vi "Configure voltage read.vi"(6 "error in":errorcluster, 8 "Range":string, 9 "VISA resource name":refnum<visa-resource-name>) -> (0 "error out":errorcluster, 3 "VISA resource name out":refnum<visa-resource-name>)   [LabVIEW 2023, in "Aim TTi 1908P DMM.lvlib"]
uses:
  Aim TTi 1908P DMM.lvlib
  34c442d0-076a-446d-8d09-49ed1551a703.vi
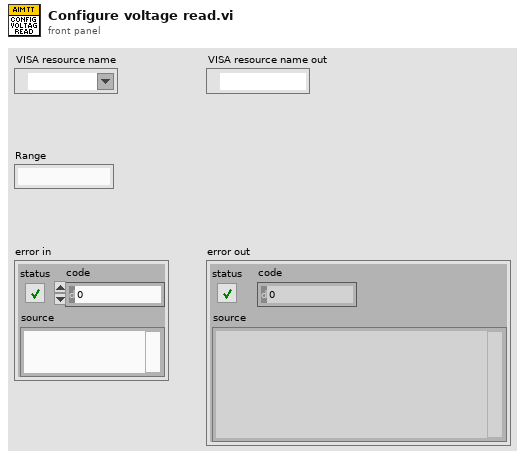
[diagram p1: front panel]
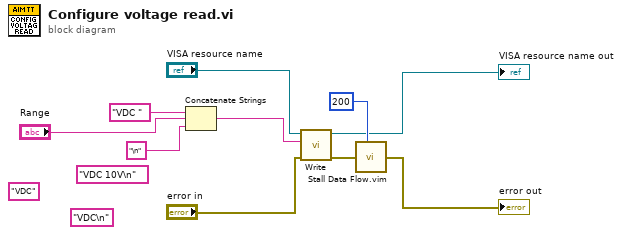
[diagram p0: block diagram]
diagram:
  (unwired) "VDC\n" ("Data to write")
  (unwired) "VDC 10V\n" ("Data to write")
  (unwired) "VDC" ("Data to write")
  n1 = Concatenate Strings("VDC " ("Data to write"), "Range", "\n" ("Data to write")) -> (w2:string)
  n2 = call "Write.vi"("error in"="error in", "Data to write"=w2, "VISA resource name"="VISA resource name") -> ("error out"=w9:errorcluster, "VISA resource name out"=→"VISA resource name out":refnum<visa-resource-name>)  [unwired: 5 in]
  n3 = call "Stall Data Flow.vim"("value in"=w9, "milliseconds to wait"=u32 200) -> ("value out"=→"error out":errorcluster)  [unwired: 1 out]
